vi "Resample Histogram.vi"(11 "AI":waveform(dbl)[](array[waveform])) -> ()   [LabVIEW 2019, in "DSP.lvclass"]
uses:
  DSP.lvclass
  <vilib>/ptbypt/NI_PtbyPt.lvlib
panel:
  out "dt Chart":dbl(graph)
  out "<Fout> S/s":dbl
  out "Histogram Graph":T1(graph)
  # "Mean rate over a long window. Count total emitted samples and divide by elapsed time - must equal #s/M S/s."
  # "t0 uniformity despite clumpy arrival. The samples arrive irregularly - sometimes two land in consecutive 0.1 s reads, sometimes there's a 0.3 s arrival gap - but their t0 timestamps must be exactly M·dt = 1716/10240 = 0.16758 s apart, dead uniform. Plot or diff the t0s of emitted samples. If anything downstream plots against arrival/loop-iteration time instead of t0, the trace will show false jitter that isn't in the data."
  # "histogram of n_out"
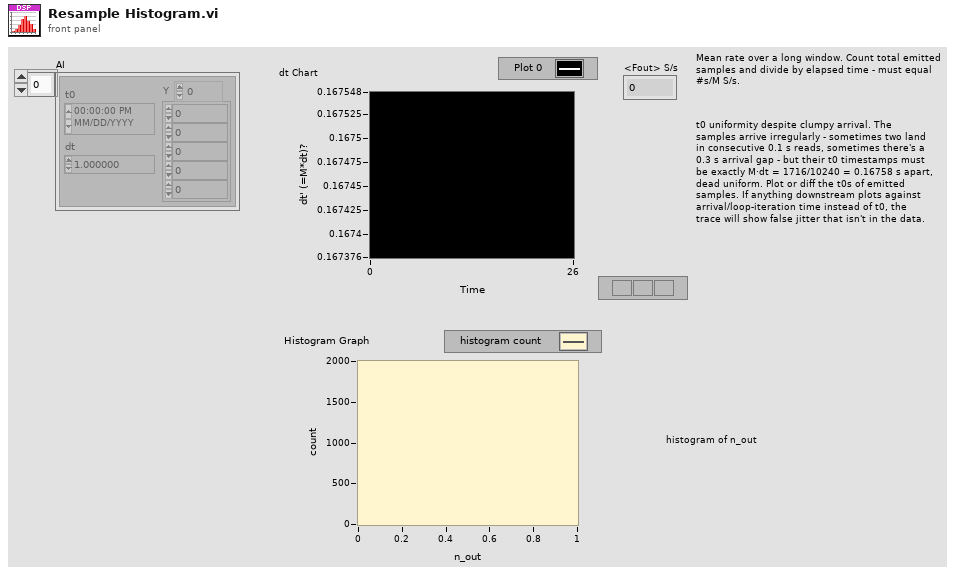
[diagram p1: front panel]
types:
  T1 = cluster{"X Values":dbl[], "Histogram: h(x)":i32[]}
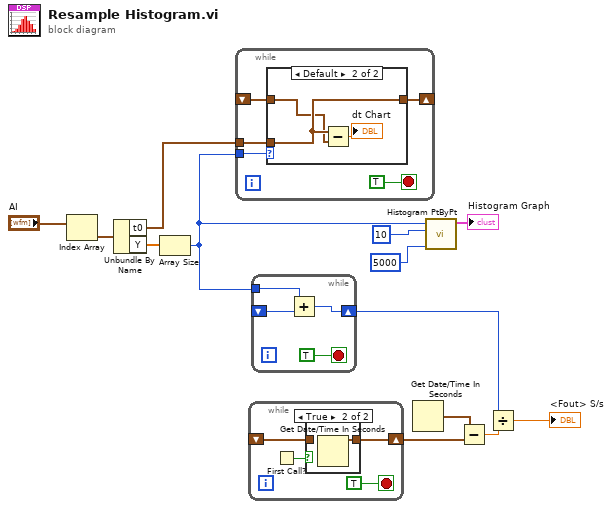
[diagram p0: block diagram]
diagram:
  n1 = Index Array(array="AI") -> (element=w1:waveform(dbl))  [unwired: 1 in]
  n2 = Unbundle By Name(w1) -> ("t0"=w11:timestamp, "Y"=w3:dbl[])
  n3 = Array Size(array=w3) -> (size(s)=w12:i32)
  n4 = while {
    tunnel: w11 -> [w15]
    shift-right: [w16] -> _
    shift-left: _ -> [w14]
    tunnel: w12 -> [w17]
    stop <- TRUE stop-if-true
    n5 = case shown="Default" w17 {
      tunnel: [w19 w22] -> w16
      tunnel: w15 -> [_ w22]
      tunnel: w14 -> [w19 w21]
      frame 0 {
      }
      frame Default {
        n6 = Subtract(x=w22, y=w21) -> (x-y=→"dt Chart":dbl)
      }
    }
  }
  n7 = while {
    shift-right: [w24] -> w6
    shift-left: _ -> [w23]
    stop <- TRUE stop-if-true
    n8 = First Call?() -> (First Call?: T/F=w25:bool)
    n9 = case shown="True" w25 {
      tunnel: [w27 w28] -> w24
      tunnel: w23 -> [w27 _]
      frame False {
      }
      frame True {
        n10 = Get Date/Time In Seconds() -> (seconds since 1Jan1904=w28:timestamp)
      }
    }
  }
  n11 = while {
    shift-right: [w31] -> w9
    shift-left: _ -> [w29]
    tunnel: w12 -> [w30]
    stop <- TRUE stop-if-true
    n12 = Add(x=w30, y=w29) -> (x+y=w31:i32)
  }
  n13 = Get Date/Time In Seconds() -> (seconds since 1Jan1904=w5:timestamp)
  n14 = call <vilib>:"Histogram PtByPt.vi"("sample length"=5000, "intervals"=10, "x"=w12) -> ("Histogram Graph"=→"Histogram Graph":T1)  [unwired: 5 in, 3 out]
  n15 = Subtract(x=w5, y=w6) -> (x-y=w7:dbl)
  n16 = Divide(x=w9, y=w7) -> (x/y=→"<Fout> S/s":dbl)
